vi "solar_cfg Read File (Ref).vi"(0 "Config Path (*.ini)":path, 1 "Section (\"\" = Use Filename)":string, 2 "Comments (Key,Comment)":cluster{"Key":string, "Comment":string}[](array[cluster]), 5 "Key_Prefix (\"\")":string, 7 "Ctrl Refnums":refnum<vi>[](array[refnum]), 11 "error in (no error)":errorcluster, 12 "ArrayDelimiters (1D,2D)":string[](array[string]), 13 "Write If Not Found? (T)":bool=TRUE) -> (4 "Config Path out":path, 10 "Found?":bool, 15 "error out":errorcluster)   [LabVIEW 2018]
doc: "Reads the values associated with a control reference from a specified section in a configuration file. If the Key is empty the control reference label is used instead. Set a Comment (#...) to add a description after the key's value. Clusters use the element lables are their key names. Set Enum as Strings to True to use the string item of an enum.\n\nSupported Data Types: \nI8..EXT, Enum, Boolean, String, Path, VISA Reference, Timestamp\n1D & 2D Arrays and Clusters of the data types above.\n\n[Section]\nKey = \"Value\" #Comment"
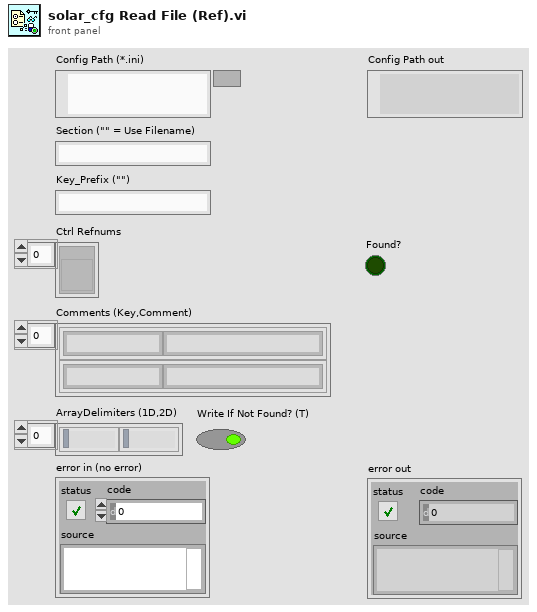
[diagram p1: front panel]
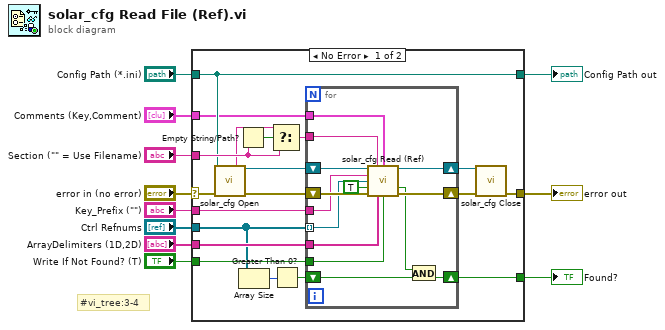
[diagram p0: block diagram]
diagram:
  # "#vi_tree:3-4"
  n1 = case shown="No Error" "error in (no error)" {
    selector: "error in (no error)" -> [w28 w46]
    tunnel: "Config Path (*.ini)" -> [w27 w45]
    tunnel: "Key_Prefix (\"\")" -> [w16 _]
    tunnel: [w19 w46] -> w8
    tunnel: "Section (\"\" = Use Filename)" -> [w29 _]
    tunnel: [w27 w45] -> w6
    tunnel: "Ctrl Refnums" -> [w15 _]
    tunnel: "Comments (Key,Comment)" -> [w24 _]
    tunnel: "ArrayDelimiters (1D,2D)" -> [w18 _]
    tunnel: "Write If Not Found? (T)" -> [w17 _]
    tunnel: [w12 _] -> w1
    frame No Error {
      n2 = call "solar_cfg Open.vi"("Config Path (*.ini)"=w27, "error in (no error)"=w28) -> ("Filename"=w26:string, "Config Refnum"=w22:refnum<data-value>, "error out"=w25:errorcluster)  [unwired: 10 in, 1 out]
      n3 = Empty String/Path?(string/path=w29) -> (empty?=w30:bool)
      n4 = Array Size(array=w15) -> (size(s)=w14:i32)
      n5 = Select(t=w26, s=w30, f=w29) -> (s? t:f=w23:string)
      n6 = Greater Than 0?(x=w14) -> (x > 0?=w13:bool)
      n7 = for {
        tunnel: w15 -> [w43] mode=indexing
        tunnel: w24 -> [w42]
        tunnel: w23 -> [w41]
        tunnel: w18 -> [w37]
        tunnel: w16 -> [w35]
        shift-right: [w38] -> w20
        shift-left: w25 -> [w44]
        shift-right: [w39] -> w21
        shift-left: w22 -> [w40]
        tunnel: w17 -> [w36]
        shift-right: [w32] -> w12
        shift-left: w13 -> [w33]
        n8 = call "solar_cfg Read (Ref).vi"("Config Refnum"=w40, "Section"=w41, "Comments (Key,Comment)"=w42, "Key_Prefix (\"\")"=w35, "Ctrl Refnum"=w43, "Update Ctrl Value? (T)"=TRUE, "error in (no error)"=w44, "ArrayDelimiters (1D,2D)"=w37, "Write If Not Found? (T)"=w36) -> ("dup Config Refnum"=w39:refnum<data-value>, "Found?"=w31:bool, "error out"=w38:errorcluster)  [unwired: 3 in, 1 out]
        n9 = And(x=w31, y=w33) -> (x .and. y?=w32:bool)
      }
      n10 = call "solar_cfg Close.vi"("Config Refnum"=w21, "error in (no error)"=w20) -> ("error out"=w19:errorcluster)  [unwired: 12 in, 1 out]
    }
    frame Error {
    }
  }
  "error out" <- w8
  "Config Path out" <- w6
  "Found?" <- w1
